vi "自动界面.vi"(8 "错误输入（无错误）":errorcluster, 10 "界面切换队列":refnum<queue>, 11 "VISA资源名称输入":refnum<visa-resource-name>) -> (0 "错误输出":errorcluster, 3 "VISA资源名称输出":refnum<visa-resource-name>)   [LabVIEW 2018]
panel:
  out "毫秒计时值":u32
  in  "枚举":T1(ring)
  in  "选项卡控件":enum32{"选项卡 1", "选项卡 2"}(tab)
  in  "报警显示":string
  out "写R2490":bool
  out "写R80":bool
  out "写R9+读R8":bool
  out "写R6+读R7":bool
  out "写R88+读R89":bool
  out "写R453":bool
  out "写R452":bool
  out "RF":bool
  out "DT1215":enum16{"关闭", "空", "烧录", "OK", "", "NG"}(ring)
  out "DT1211":enum16{"关闭", "空", "烧录", "OK", "", "NG"}(ring)
  out "DT1207":enum16{"关闭", "空", "烧录", "OK", "", "NG"}(ring)
  out "DT1203":enum16{"关闭", "空", "烧录", "OK", "", "NG"}(ring)
  out "DT1214":enum16{"关闭", "空", "烧录", "OK", "", "NG"}(ring)
  out "DT1210":enum16{"关闭", "空", "烧录", "OK", "", "NG"}(ring)
  out "DT1206":enum16{"关闭", "空", "烧录", "OK", "", "NG"}(ring)
  out "DT1202":enum16{"关闭", "空", "烧录", "OK", "", "NG"}(ring)
  out "DT1213":enum16{"关闭", "空", "烧录", "OK", "", "NG"}(ring)
  out "DT1209":enum16{"关闭", "空", "烧录", "OK", "", "NG"}(ring)
  out "DT1205":enum16{"关闭", "空", "烧录", "OK", "", "NG"}(ring)
  out "DT1201":enum16{"关闭", "空", "烧录", "OK", "", "NG"}(ring)
  out "DT1212":enum16{"关闭", "空", "烧录", "OK", "", "NG"}(ring)
  out "DT1208":enum16{"关闭", "空", "烧录", "OK", "", "NG"}(ring)
  out "DT1204":enum16{"关闭", "空", "烧录", "OK", "", "NG"}(ring)
  out "DT1200":enum16{"关闭", "空", "烧录", "OK", "", "NG"}(ring)
  out "R77":bool
  out "R76":bool
  out "R75":bool
  out "DT776":dbl
  out "DT770":dbl
  out "DT676":dbl
  out "DT670":dbl
  out "DT666":dbl
  out "DT660":dbl
  out "DDT594":dbl
  out "DDT604":dbl
  out "DDT600":dbl
  out "DDT590":dbl
  out "DDT32700":dbl
  out "DDT32750":dbl
  out "DDT32748":dbl
  out "DT1000+6位":string
  out "DT32622":dbl
  out "DDT90356":dbl
  out "DDT90348":dbl
  out "自动界面":bool
  out "手动界面":bool
  out "参数界面":bool
  out "IO界面":bool
  out "产品界面":bool
  out "字符串":string
  out "DDT90352":dbl
  out "DDT90360":dbl
  out "XC":bool
  out "写R454":bool
  out "写R2+读R3":bool
  out "写R87":bool
  out "通讯周期":dbl
  out "DT1184":T2(ring)
  # "X"
  # "Z1"
  # "Z2"
  # "Y"
  # "设定产量"
  # "当前产品"
  # "当前产量"
  # "NG产量"
  # "烧录座状态"
  # "修改"
  # "已取"
  # "行数"
  # "列数"
  # "已放"
  # "04"
  # "03"
  # "主料盘"
  # "02"
  # "01"
  # "08"
  # "07"
  # "05"
  # "06"
  # "备料盘"
  # "12"
  # "11"
  # "09"
  # "10"
  # "废料盘"
  # "14"
  # "15"
  # "13"
  # "14"
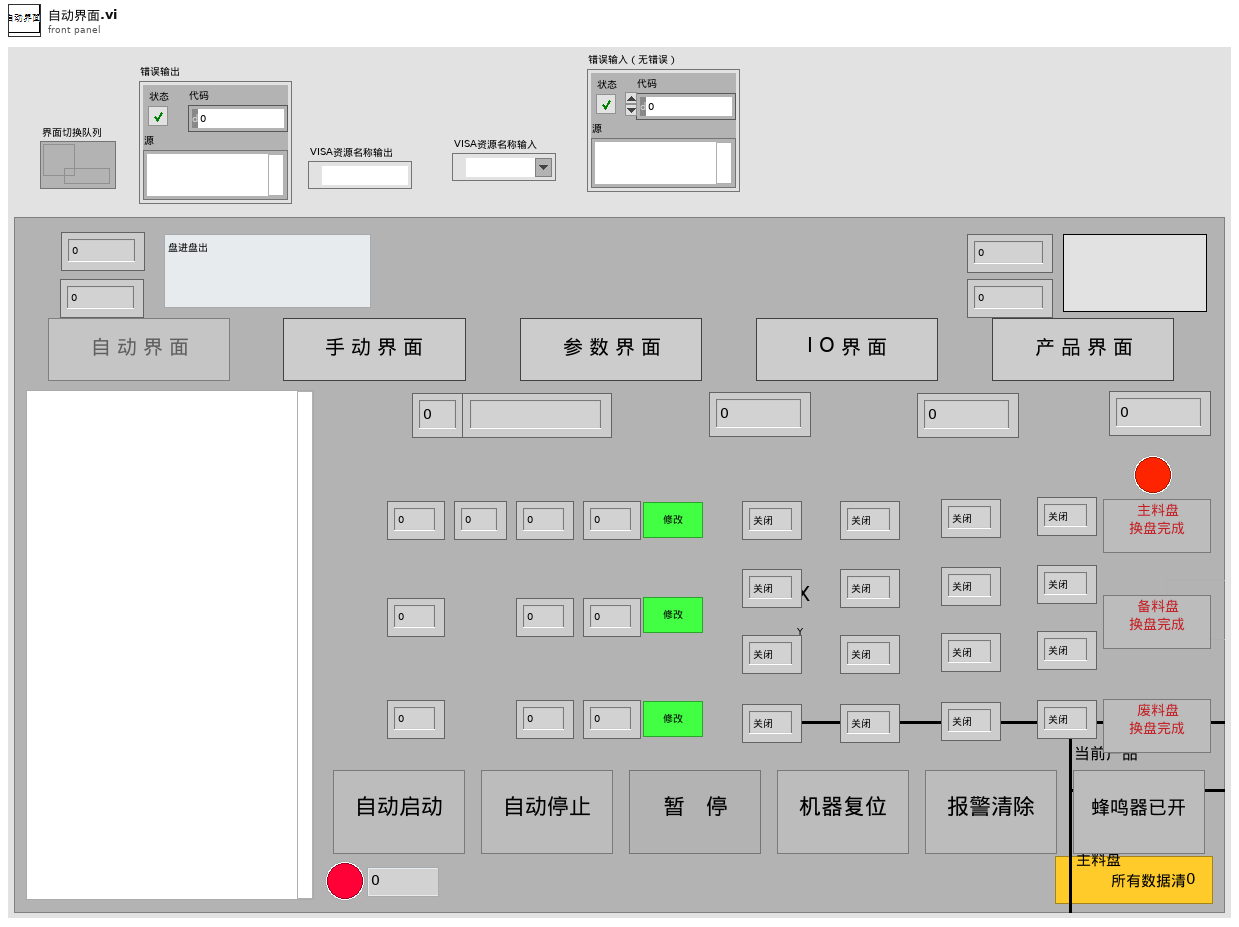
[diagram p1: front panel]
types:
  T1 = enum16{"读初始化", "读R598+8+报警", "读R590+8+报警", "读R588+8+报警", "读R580+8+报警", "读R405+8+报警", "读R410+8+报警", "读R221+8+报警", "读R449+8+报警", "读R450+8+报警", "读R441+8+报警", "读R89+8+报警", "读R72+8+报警", "读X1C+8+报警", "读R400+8+报警", "读T700+8+报警", "读X8+8+报警", "读R80+8", "读RF+8", "读XC+8", "读R2490+8", "读R452+8", "读R87+8", "读R75+8", "读R2+8", "读DDT90356", "读DT1184", "读DT1000+6", "读DT1210+10", "读DT1200+10", "读DT770", "读DT32622", "无", "读DDT32700", "读DDT32750+10", "读DT670+10", "读DT660+10", "读DDT600+10", "读DDT590+10", "读DDT90348", ""}
  T2 = enum16{"盘进盘出", "卷进卷出", "盘进卷出", "管进盘出", "管进卷出", "卷进盘出", ""}
  T3 = enum8{"Enabled", "Disabled", "Disabled and Grayed Out"}
  T4 = typedef "数据簇.ctl" = cluster{"字符串":string, "数值":i32, "布尔":bool}
  T5 = typedef "lveventtype.ctl" = enum32{"Null", "Timeout", "Annotation Menu Selection", "Annotation Menu Selection?", "App Instance Close", "App Instance Close?", "Autoscale Range Change", "Bookmark Info Change", "Cell Edit", "Cell Edit?", "Cursor Grab", "Cursor Grab?", "Cursor Menu Selection", "Cursor Menu Selection?", "Cursor Move", "Cursor Release", "Data Change", "Direction Change", "Display State Change", "Drag Ended", "Drag Enter", "Drag Leave", "Drag Over", "Drag Source Update", "Drag Starting", "Drag Starting?", "Drop", "Exec State Change", "Key Down", "Key Down?", "Key Repeat", "Key Repeat?", "Key Up", "Listbox Double Click", "Menu Activation?", "Menu Selection (App)", "Menu Selection? (App)", "Menu Selection (User)", "Mouse Down", "Mouse Down?", "Mouse Enter", "Mouse Leave", "Mouse Move", "Mouse Up", "Mouse Wheel", "NI Security User Change (App)", "Pane Size", "Panel Close", "Panel Close?", "Panel Resize", "Plot Attribute Change", "Scale Range Change", "Shortcut Menu Activation?", "Shortcut Menu Selection (App)", "Shortcut Menu Selection? (App)", "Shortcut Menu Selection (User)", "Tree Double Click", "Tree Drag", "Tree Drag?", "Tree Drop", "Tree Drop?", "Tree Item Close", "Tree Item Close?", "Tree Item Open", "Tree Item Open?", "User Event", "Value Change"}
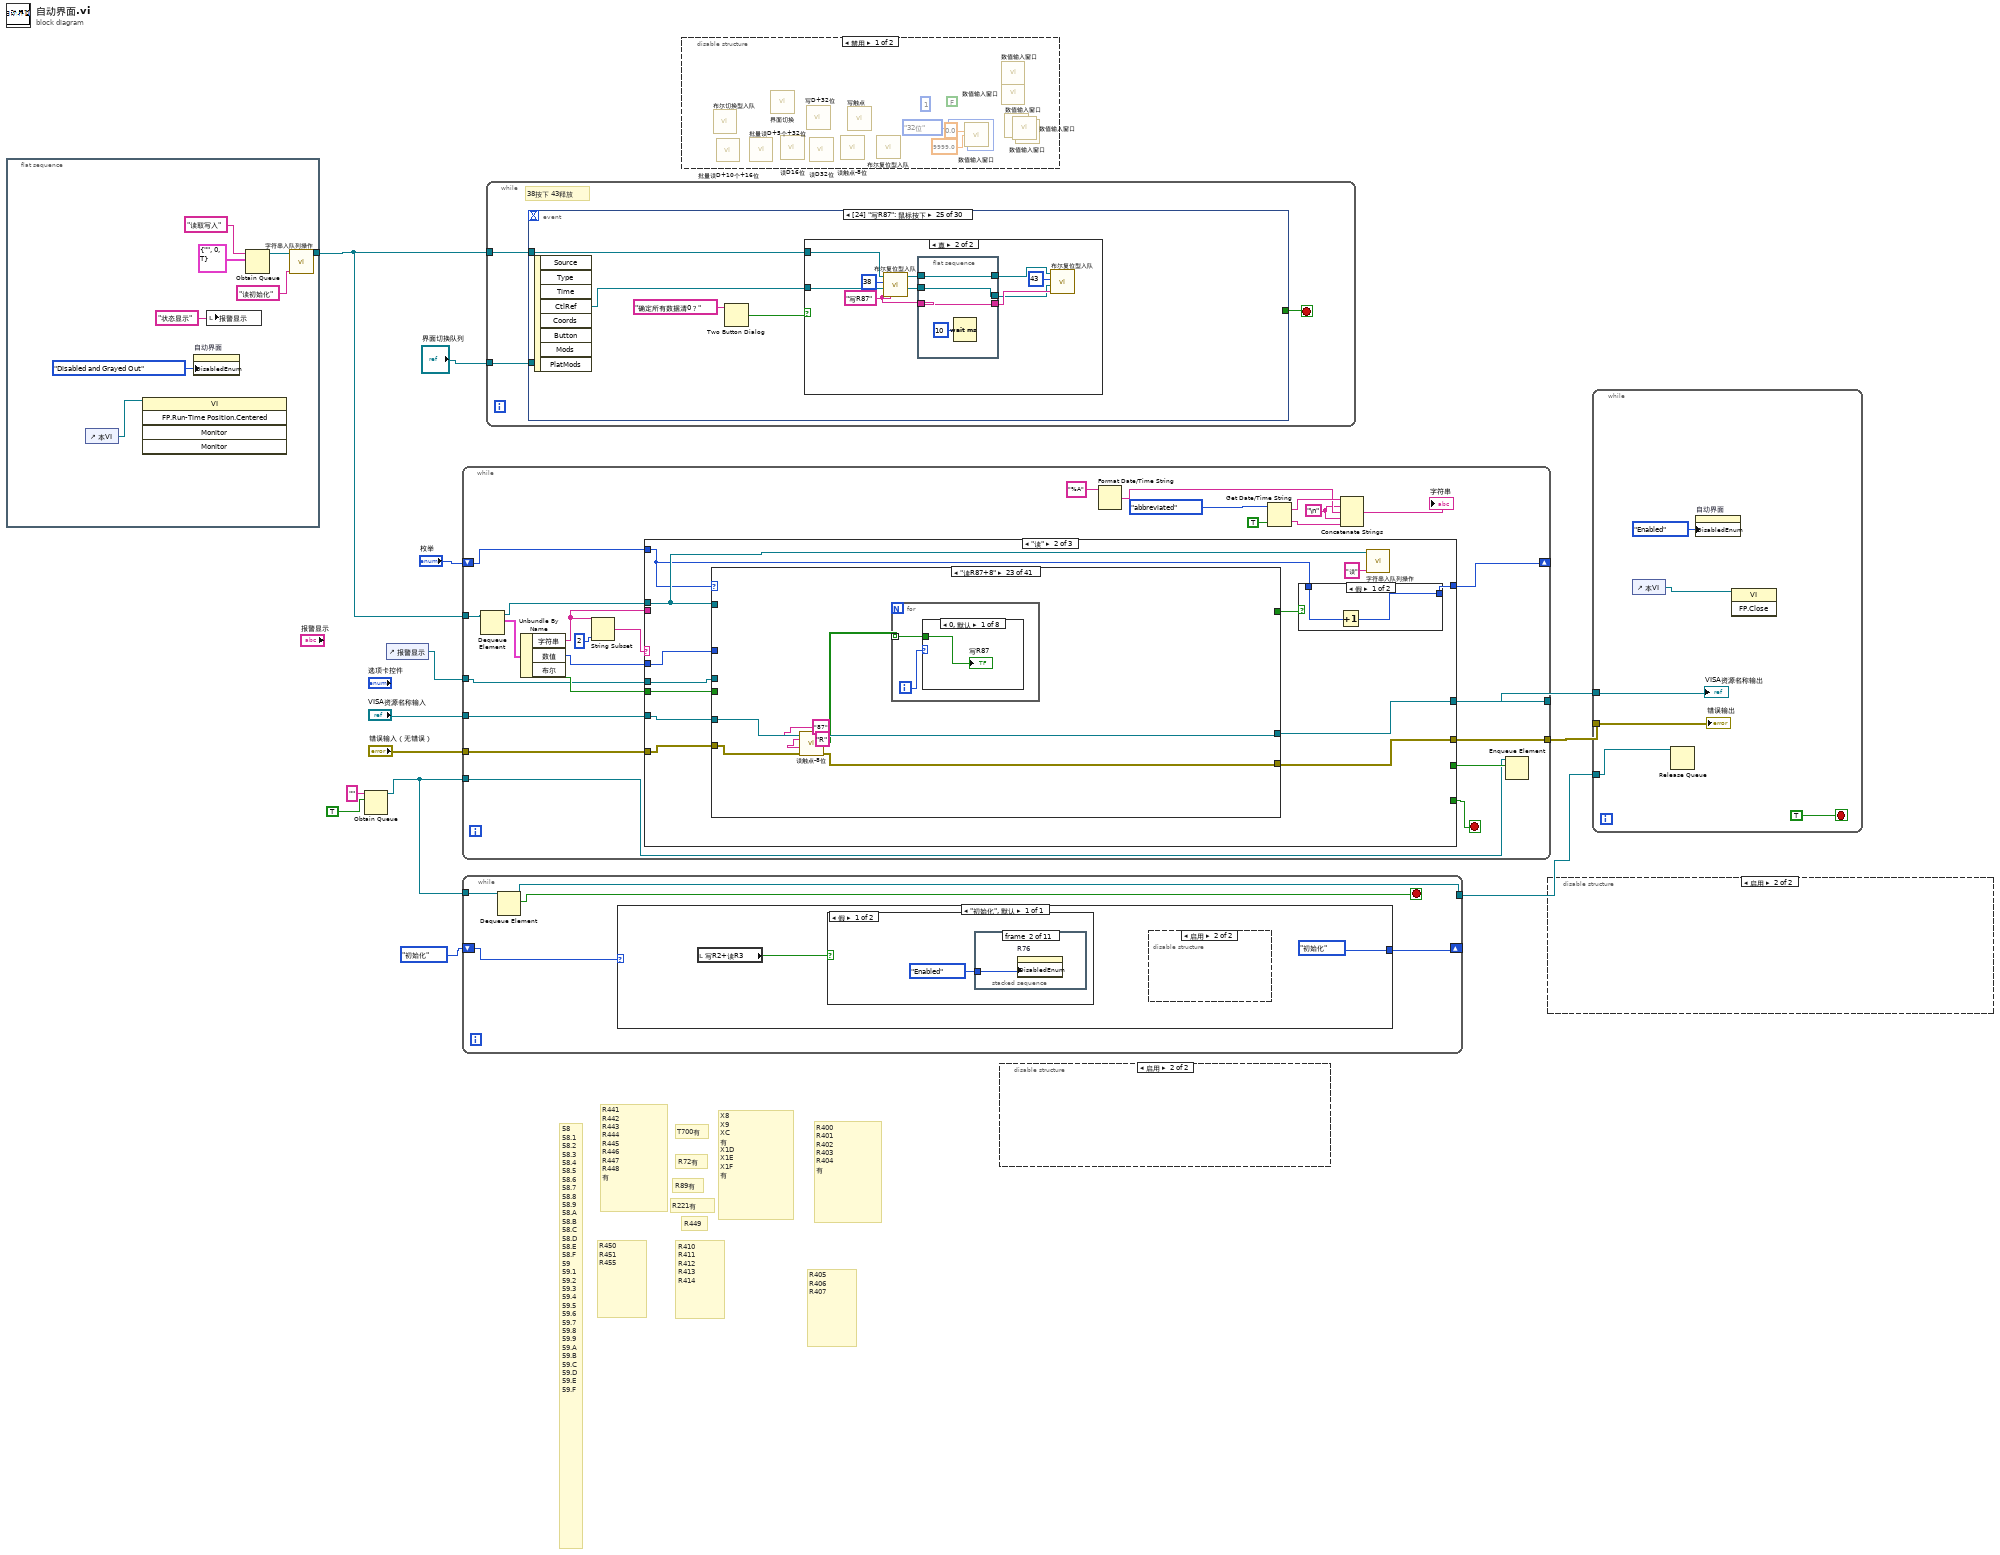
[diagram p0: block diagram]
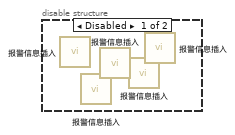
[diagram p2: hidden frame]
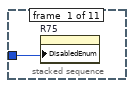
[diagram p3: hidden frame]
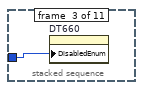
[diagram p4: hidden frame]
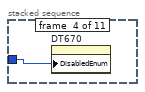
[diagram p5: hidden frame]
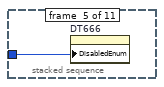
[diagram p6: hidden frame]
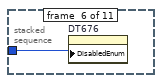
[diagram p7: hidden frame]
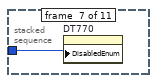
[diagram p8: hidden frame]
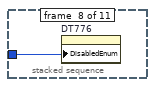
[diagram p9: hidden frame]
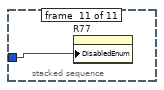
[diagram p12: hidden frame]
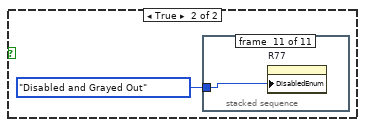
[diagram p13: hidden frame]
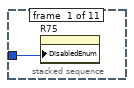
[diagram p14: hidden frame]
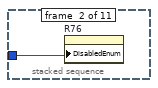
[diagram p15: hidden frame]
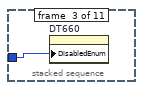
[diagram p16: hidden frame]
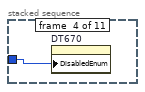
[diagram p17: hidden frame]
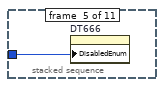
[diagram p18: hidden frame]
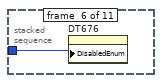
[diagram p19: hidden frame]
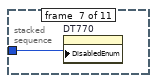
[diagram p20: hidden frame]
diagram:
  # "R449"
  # "R405\nR406\nR407"
  # "R410\nR411\nR412\nR413\nR414"
  # "R221有"
  # "R89有"
  # "R450\nR451\nR455"
  # "R72有"
  # "R441\nR442\nR443\nR444\nR445\nR446\nR447\nR448\n有"
  # "R400\nR401\nR402\nR403\nR404\n有"
  # "T700有"
  # "X8\nX9\nXC\n有\nX1D\nX1E\nX1F\n有"
  # "58\n58.1\n58.2\n58.3\n58.4\n58.5\n58.6\n58.7\n58.8\n58.9\n58.A\n58.B\n58.C\n58.D\n58.E\n58.F\n59\n59.1\n59.2\n59.3\n59.4\n59.5\n59.6\n59.7\n59.8\n59.9\n59.A\n59.B\n59.C\n59.D\n59.E\n59.F"
  n1 = flat-sequence {
    tunnel: [w21] -> w2
    frame #0 {
      n2 = control-ref of="本VI"() -> (w14:refnum<vi>)
      n3 = invoke class="VI" method="FP.Run-Time Position.Centered"(reference=w14) -> ()  [unwired: 4 in, 5 out]
      n4 = property on="自动界面" class="Bool"("DisabledEnum"=T3."Disabled and Grayed Out" ("禁用")) -> ()  [unwired: 2 in, 2 out]
      n5 = local write "报警显示"("状态显示") -> ()
      n6 = Obtain Queue(name (unnamed)="读取写入" ("名称（未命名）"), element data type=T4 {"字符串"="", "数值"=0, "布尔"=TRUE}) -> (queue out=w17:refnum<queue>)  [unwired: 3 in, 2 out]
      n7 = call "字符串入队列操作.vi"("字符消息入队列"="读初始化", "界面切换队列"=w17) -> ("队列输出"=w21:refnum<queue>)  [unwired: 9 in]
    }
  }
  n8 = Obtain Queue(name (unnamed)="" ("名称（未命名）"), element data type=TRUE) -> (queue out=w6:refnum<queue>)  [unwired: 3 in, 2 out]
  n9 = control-ref of="报警显示"() -> (w4:refnum<vi>)
  n10 = while {
    tunnel: w2 -> [w43]
    tunnel: "VISA资源名称输入" -> [w36]
    tunnel: "错误输入（无错误）" -> [w35]
    tunnel: [w34] -> w11
    tunnel: [w33] -> w10
    shift-right: [w30] -> _
    shift-left: "枚举" -> [w31]
    tunnel: w6 -> [w23]
    tunnel: w4 -> [w22]
    stop <- w25 stop-if-true
    w27 = "\n"
    n11 = Dequeue Element(queue=w43) -> (queue out=w40:refnum<queue>, element=w42:T4)  [unwired: 2 in, 2 out]
    n12 = Unbundle By Name(w42) -> ("字符串"=w37:string, "数值"=w39:i32, "布尔"=w38:bool)
    n13 = String Subset(string=w37, length (rest)=2 ("长度（剩余）")) -> (substring=w41:string)  [unwired: 1 in]
    n14 = case shown="\"读\"" w41 {
      selector: w41 -> [w50 _ _]
      tunnel: w40 -> [_ w59 w800]
      tunnel: w39 -> [_ w66 w799]
      tunnel: w38 -> [_ w65 w798]
      tunnel: w37 -> [_ _ w792]
      tunnel: w36 -> [w49 w64 w797]
      tunnel: w35 -> [w48 w63 w796]
      tunnel: [w49 w62 w794] -> w34
      tunnel: [w48 w61 w793] -> w33
      tunnel: [_ _ w795] -> w25
      tunnel: w31 -> [_ w57 _]
      tunnel: [_ w56 _] -> w30
      tunnel: [_ _ w790] -> w24
      tunnel: w22 -> [_ w55 _]
      frame "", Default {
        n15 = Concatenate Strings("无对应消息分支**" ("消息"), w50, "**" ("字符串"), "读写状态机" ("字符串")) -> (w52:string)
        n16 = One Button Dialog(message=w52) -> ()  [unwired: 1 in, 1 out]
      }
      frame "读" {
        n17 = case shown="\"读R87+8\"" w57 {
          tunnel: w59 -> [_ _ _ _ _ _ _ _ _ _ _ _ _ _ _ _ _ _ _ _ _ _ _ _ _ _ _ _ _ _ _ _ _ _ _ _ _ _ _ _ _]
          tunnel: w66 -> [_ _ _ _ _ _ _ _ _ _ _ _ _ _ _ _ _ _ _ _ _ _ _ _ _ _ _ _ _ _ _ _ _ _ _ _ _ _ _ _ _]
          tunnel: w64 -> [w71 w79 w117 w155 w193 w225 w236 w262 w284 w306 w330 w359 w381 w403 w431 w460 w491 w524 w534 w545 w556 w566 w578 w589 w601 w618 w627 w636 w665 w679 w697 w707 w709 w715 w721 w731 w741 w751 w761 w777 w789]
          tunnel: w63 -> [w70 w78 w116 w154 w192 w224 w235 w261 w283 w305 w329 w358 w380 w402 w430 w459 w490 w523 w533 w544 w555 w565 w577 w588 w600 w617 w626 w635 w664 w678 w696 w706 w708 w714 w720 w730 w740 w750 w760 w776 w788]
          tunnel: [w71 w75 w113 w151 w191 w225 w234 w260 w282 w304 w326 w355 w377 w399 w429 w456 w489 w520 w532 w541 w552 w562 w574 w585 w597 w616 w625 w629 w662 w676 w694 w704 w709 w712 w718 w728 w738 w749 w758 w775 w789] -> w62
          tunnel: [w70 w74 w112 w150 w190 w224 w233 w259 w281 w303 w325 w354 w376 w398 w428 w455 w488 w519 w531 w540 w551 w561 w573 w584 w596 w615 w624 w631 w661 w675 w693 w703 w708 w711 w717 w727 w737 w748 w757 w774 w788] -> w61
          tunnel: w65 -> [_ _ _ _ _ _ _ _ _ _ _ _ _ _ _ _ _ _ _ _ _ _ _ _ _ _ _ _ _ _ _ _ _ _ _ _ _ _ _ _ _]
          tunnel: [_ _ _ _ _ _ _ _ _ _ _ _ _ _ _ _ _ _ _ _ _ _ _ _ _ _ _ _ _ _ _ _ _ _ _ _ _ _ _ _ TRUE] -> w58
          tunnel: w55 -> [_ w72 w110 w148 w186 _ w229 w255 w277 w299 w323 w352 w374 w396 w424 w453 w484 _ _ w538 _ _ _ _ _ _ _ _ _ _ _ _ _ _ _ _ _ _ _ _ _]
          frame "读初始化" {
            n18 = Tick Count (ms)() -> (millisecond timer value=→"毫秒计时值":u32)
          }
          frame "读R598+8+报警" {
            n19 = call "读触点-8位.vi"("error out"=w78, "触点类型"="R", "读取起始地址"="598", "VISA resource name out"=w79) -> ("error IO"=w74:errorcluster, "读取布尔数组"=w73:bool[], "VISA resource name out 2"=w75:refnum<visa-resource-name>)  [unwired: 4 in, 1 out]
            n20 = for {
              tunnel: w73 -> [w84] mode=indexing
              tunnel: w72 -> [w83]
              i -> [w85]
              n21 = case shown="7" w85 {
                tunnel: w84 -> [w87 w90 w93 w96 w99 w102 w105 w108]
                tunnel: w83 -> [w88 w91 w94 w97 w100 w103 w106 w109]
                tunnel: [w88 w91 w94 w97 w100 w103 w106 w109] -> w82
                tunnel: [w87 w90 w93 w96 w99 w102 w105 w108] -> w81
                tunnel: ["9#烧录座连续NG超过设定的次数" "10#烧录座连续NG超过设定的次数" "11#烧录座连续NG超过设定的次数" "12#烧录座连续NG超过设定的次数" "13#烧录座连续NG超过设定的次数" "14#烧录座连续NG超过设定的次数" "15#烧录座连续NG超过设定的次数" "16#烧录座连续NG超过设定的次数"] -> w80
                frame 0, Default {
                }
                frame 1 {
                }
                frame 2 {
                }
                frame 3 {
                }
                frame 4 {
                }
                frame 5 {
                }
                frame 6 {
                }
                frame 7 {
                }
              }
              n22 = call "报警信息插入.vi"("输入字符串"=w80, "布尔"=w81, "Str引用句柄"=w82) -> ()  [unwired: 4 in, 1 out]
            }
          }
          frame "读R590+8+报警" {
            n23 = call "读触点-8位.vi"("error out"=w116, "触点类型"="R", "读取起始地址"="590", "VISA resource name out"=w117) -> ("error IO"=w112:errorcluster, "读取布尔数组"=w111:bool[], "VISA resource name out 2"=w113:refnum<visa-resource-name>)  [unwired: 4 in, 1 out]
            n24 = for {
              tunnel: w111 -> [w122] mode=indexing
              tunnel: w110 -> [w121]
              i -> [w123]
              n25 = case shown="7" w123 {
                tunnel: w122 -> [w125 w129 w131 w134 w137 w140 w143 w146]
                tunnel: w121 -> [w124 w128 w132 w135 w138 w141 w144 w147]
                tunnel: ["1#烧录座连续NG超过设定的次数" ("输入字符串") "2#烧录座连续NG超过设定的次数" ("输入字符串") "3#烧录座连续NG超过设定的次数" ("输入字符串") "4#烧录座连续NG超过设定的次数" ("输入字符串") "5#烧录座连续NG超过设定的次数" ("输入字符串") "6#烧录座连续NG超过设定的次数" ("输入字符串") "7#烧录座连续NG超过设定的次数" ("输入字符串") "8#烧录座连续NG超过设定的次数" ("输入字符串")] -> w120
                tunnel: [w125 w129 w131 w134 w137 w140 w143 w146] -> w119
                tunnel: [w124 w128 w132 w135 w138 w141 w144 w147] -> w118
                frame 0, Default {
                }
                frame 1 {
                }
                frame 2 {
                }
                frame 3 {
                }
                frame 4 {
                }
                frame 5 {
                }
                frame 6 {
                }
                frame 7 {
                }
              }
              n26 = call "报警信息插入.vi"("输入字符串"=w120, "布尔"=w119, "Str引用句柄"=w118) -> ()  [unwired: 4 in, 1 out]
            }
          }
          frame "读R588+8+报警" {
            n27 = call "读触点-8位.vi"("error out"=w154, "触点类型"="R", "读取起始地址"="588", "VISA resource name out"=w155) -> ("error IO"=w150:errorcluster, "读取布尔数组"=w149:bool[], "VISA resource name out 2"=w151:refnum<visa-resource-name>)  [unwired: 4 in, 1 out]
            n28 = for {
              tunnel: w149 -> [w160] mode=indexing
              tunnel: w148 -> [w159]
              i -> [w161]
              n29 = case shown="7" w161 {
                tunnel: w160 -> [w163 w166 w169 w172 w175 w178 w181 w184]
                tunnel: w159 -> [w164 w167 w170 w173 w176 w179 w182 w185]
                tunnel: [w164 w167 w170 w173 w176 w179 w182 w185] -> w158
                tunnel: [w163 w166 w169 w172 w175 w178 w181 w184] -> w157
                tunnel: ["9#烧录座到达设的的使用寿命" "10#烧录座到达设的的使用寿命" "11#烧录座到达设的的使用寿命" "12#烧录座到达设的的使用寿命" "13#烧录座到达设的的使用寿命" "14#烧录座到达设的的使用寿命" "15#烧录座到达设的的使用寿命" "16#烧录座到达设的的使用寿命"] -> w156
                frame 0, Default {
                }
                frame 1 {
                }
                frame 2 {
                }
                frame 3 {
                }
                frame 4 {
                }
                frame 5 {
                }
                frame 6 {
                }
                frame 7 {
                }
              }
              n30 = call "报警信息插入.vi"("输入字符串"=w156, "布尔"=w157, "Str引用句柄"=w158) -> ()  [unwired: 4 in, 1 out]
            }
          }
          frame "读R580+8+报警" {
            n31 = call "读触点-8位.vi"("error out"=w192, "触点类型"="R", "读取起始地址"="580", "VISA resource name out"=w193) -> ("error IO"=w190:errorcluster, "读取布尔数组"=w187:bool[], "VISA resource name out 2"=w191:refnum<visa-resource-name>)  [unwired: 4 in, 1 out]
            n32 = for {
              tunnel: w187 -> [w198] mode=indexing
              tunnel: w186 -> [w197]
              i -> [w199]
              n33 = case shown="7" w199 {
                tunnel: w198 -> [w201 w204 w207 w210 w213 w216 w219 w222]
                tunnel: w197 -> [w202 w205 w208 w211 w214 w217 w220 w223]
                tunnel: [w202 w205 w208 w211 w214 w217 w220 w223] -> w196
                tunnel: [w201 w204 w207 w210 w213 w216 w219 w222] -> w195
                tunnel: ["1#烧录座到达设的的使用寿命" "2#烧录座到达设的的使用寿命" "3#烧录座到达设的的使用寿命" "4#烧录座到达设的的使用寿命" "5#烧录座到达设的的使用寿命" "6#烧录座到达设的的使用寿命" "7#烧录座到达设的的使用寿命" "8#烧录座到达设的的使用寿命"] -> w194
                frame 0, Default {
                }
                frame 1 {
                }
                frame 2 {
                }
                frame 3 {
                }
                frame 4 {
                }
                frame 5 {
                }
                frame 6 {
                }
                frame 7 {
                }
              }
              n34 = call "报警信息插入.vi"("输入字符串"=w194, "布尔"=w195, "Str引用句柄"=w196) -> ()  [unwired: 4 in, 1 out]
            }
          }
          frame "读R405+8+报警" {
            n35 = disable-structure shown="禁用" {
              frame Disabled {
                (unwired) "R" ("触点类型")
                n36 = call "读触点-8位.vi"("读取起始地址"="405") -> ()  [unwired: 7 in, 4 out]
                n37 = for {
                  tunnel: _ -> [w227] mode=indexing
                  i -> [w228]
                  n38 = case shown="7" w228 {
                    tunnel: w227 -> [_ _ _ _ _ _ _ _]
                    frame 0, Default {
                    }
                    frame 1 {
                    }
                    frame 2 {
                    }
                    frame 3 {
                    }
                    frame 4 {
                    }
                    frame 5 {
                    }
                    frame 6 {
                    }
                    frame 7 {
                    }
                  }
                }
              }
              frame Enabled {
              }
            }
          }
          frame "读R410+8+报警" {
            n39 = call "读触点-8位.vi"("error out"=w235, "触点类型"="R", "读取起始地址"="410", "VISA resource name out"=w236) -> ("error IO"=w233:errorcluster, "读取布尔数组"=w230:bool[], "VISA resource name out 2"=w234:refnum<visa-resource-name>)  [unwired: 4 in, 1 out]
            n40 = for {
              tunnel: w230 -> [w240] mode=indexing
              tunnel: w229 -> [w239]
              i -> [w241]
              n41 = case shown="4" w241 {
                tunnel: w240 -> [w243 w245 w247 w249 w251 w252 w253 w254]
                tunnel: [w243 w245 w247 w249 w251 w252 w253 w254] -> w238
                tunnel: ["请给管道加料！" "X轴极限报警" "Y轴极限报警" "Z1轴极限报警" "Z2轴极限报警" _ _ _] -> w237
                frame 0, Default {
                }
                frame 1 {
                }
                frame 2 {
                }
                frame 3 {
                }
                frame 4 {
                }
                frame 5 {
                }
                frame 6 {
                }
                frame 7 {
                }
              }
              n42 = call "报警信息插入.vi"("输入字符串"=w237, "布尔"=w238, "Str引用句柄"=w239) -> ()  [unwired: 4 in, 1 out]
            }
          }
          frame "读R221+8+报警" {
            n43 = call "读触点-8位.vi"("error out"=w261, "触点类型"="R", "读取起始地址"="221", "VISA resource name out"=w262) -> ("error IO"=w259:errorcluster, "读取布尔数组"=w256:bool[], "VISA resource name out 2"=w260:refnum<visa-resource-name>)  [unwired: 4 in, 1 out]
            n44 = for {
              tunnel: w256 -> [w266] mode=indexing
              tunnel: w255 -> [w265]
              i -> [w267]
              n45 = case shown="0, 默认" w267 {
                tunnel: w266 -> [w269 w270 w271 w272 w273 w274 w275 w276]
                tunnel: [w269 w270 w271 w272 w273 w274 w275 w276] -> w264
                tunnel: ["正在待机！" _ _ _ _ _ _ _] -> w263
                frame 0, Default {
                }
                frame 1 {
                }
                frame 2 {
                }
                frame 3 {
                }
                frame 4 {
                }
                frame 5 {
                }
                frame 6 {
                }
                frame 7 {
                }
              }
              n46 = call "报警信息插入.vi"("输入字符串"=w263, "布尔"=w264, "Str引用句柄"=w265) -> ()  [unwired: 4 in, 1 out]
            }
          }
          frame "读R449+8+报警" {
            n47 = call "读触点-8位.vi"("error out"=w283, "触点类型"="R", "读取起始地址"="449", "VISA resource name out"=w284) -> ("error IO"=w281:errorcluster, "读取布尔数组"=w278:bool[], "VISA resource name out 2"=w282:refnum<visa-resource-name>)  [unwired: 4 in, 1 out]
            n48 = for {
              tunnel: w278 -> [w288] mode=indexing
              tunnel: w277 -> [w287]
              i -> [w289]
              n49 = case shown="0, 默认" w289 {
                tunnel: w288 -> [w291 w292 w293 w294 w295 w296 w297 w298]
                tunnel: [w291 w292 w293 w294 w295 w296 w297 w298] -> w286
                tunnel: ["没有收到卷带收料完成信号！R449" _ _ _ _ _ _ _] -> w285
                frame 0, Default {
                }
                frame 1 {
                }
                frame 2 {
                }
                frame 3 {
                }
                frame 4 {
                }
                frame 5 {
                }
                frame 6 {
                }
                frame 7 {
                }
              }
              n50 = call "报警信息插入.vi"("输入字符串"=w285, "布尔"=w286, "Str引用句柄"=w287) -> ()  [unwired: 4 in, 1 out]
            }
          }
          frame "读R450+8+报警" {
            n51 = call "读触点-8位.vi"("error out"=w305, "触点类型"="R", "读取起始地址"="450", "VISA resource name out"=w306) -> ("error IO"=w303:errorcluster, "读取布尔数组"=w300:bool[], "VISA resource name out 2"=w304:refnum<visa-resource-name>)  [unwired: 4 in, 1 out]
            n52 = for {
              tunnel: w300 -> [w310] mode=indexing
              tunnel: w299 -> [w309]
              i -> [w311]
              n53 = case shown="7" w311 {
                tunnel: w310 -> [w313 w315 w316 w317 w318 w320 w321 w322]
                tunnel: [w313 w315 w316 w317 w318 w320 w321 w322] -> w308
                tunnel: ["已完成设定的编带数量，要再次启动，请先将已完成数量清零！" "备料盘已取完，请更换备料盘，然后点击备料盘更换完成！" _ _ _ "NG数量到达提示数量，请注意！" _ _] -> w307
                frame 0, Default {
                }
                frame 1 {
                }
                frame 2 {
                }
                frame 3 {
                }
                frame 4 {
                }
                frame 5 {
                }
                frame 6 {
                }
                frame 7 {
                }
              }
              n54 = call "报警信息插入.vi"("输入字符串"=w307, "布尔"=w308, "Str引用句柄"=w309) -> ()  [unwired: 4 in, 1 out]
            }
          }
          frame "读R441+8+报警" {
            n55 = call "读触点-8位.vi"("error out"=w329, "触点类型"="R", "读取起始地址"="441", "VISA resource name out"=w330) -> ("error IO"=w325:errorcluster, "读取布尔数组"=w324:bool[], "VISA resource name out 2"=w326:refnum<visa-resource-name>)  [unwired: 4 in, 1 out]
            n56 = for {
              tunnel: w324 -> [w334] mode=indexing
              tunnel: w323 -> [w333]
              i -> [w335]
              n57 = case shown="1" w335 {
                tunnel: w334 -> [w337 w339 w341 w343 w345 w347 w349 w351]
                tunnel: [w337 w339 w341 w343 w345 w347 w349 w351] -> w332
                tunnel: ["生产模式时没收到自动换盘完成信号，不能启动！" "正在等待换盘完成！" "主料盘数量不能为0，请修改参数！" "备料盘数量不能为0，请修改参数！" "废料盘数量不能为0，请修改参数！" "废料盘已放满，请更换废料盘，然后点击废料盘更换完成！" "正在等待换盘！" "没有收到卷带收料完成信号！R448"] -> w331
                frame 0, Default {
                }
                frame 1 {
                }
                frame 2 {
                }
                frame 3 {
                }
                frame 4 {
                }
                frame 5 {
                }
                frame 6 {
                }
                frame 7 {
                }
              }
              n58 = call "报警信息插入.vi"("输入字符串"=w331, "布尔"=w332, "Str引用句柄"=w333) -> ()  [unwired: 4 in, 1 out]
            }
          }
          frame "读R89+8+报警" {
            n59 = call "读触点-8位.vi"("error out"=w358, "触点类型"="R", "读取起始地址"="89", "VISA resource name out"=w359) -> ("error IO"=w354:errorcluster, "读取布尔数组"=w353:bool[], "VISA resource name out 2"=w355:refnum<visa-resource-name>)  [unwired: 4 in, 1 out]
            n60 = for {
              tunnel: w353 -> [w363] mode=indexing
              tunnel: w352 -> [w362]
              i -> [w364]
              n61 = case shown="0, 默认" w364 {
                tunnel: w363 -> [w366 w367 w368 w369 w370 w371 w372 w373]
                tunnel: [w366 w367 w368 w369 w370 w371 w372 w373] -> w361
                tunnel: ["正在准备停机！" _ _ _ _ _ _ _] -> w360
                frame 0, Default {
                }
                frame 1 {
                }
                frame 2 {
                }
                frame 3 {
                }
                frame 4 {
                }
                frame 5 {
                }
                frame 6 {
                }
                frame 7 {
                }
              }
              n62 = call "报警信息插入.vi"("输入字符串"=w360, "布尔"=w361, "Str引用句柄"=w362) -> ()  [unwired: 4 in, 1 out]
            }
          }
          frame "读R72+8+报警" {
            n63 = call "读触点-8位.vi"("error out"=w380, "触点类型"="R", "读取起始地址"="72", "VISA resource name out"=w381) -> ("error IO"=w376:errorcluster, "读取布尔数组"=w375:bool[], "VISA resource name out 2"=w377:refnum<visa-resource-name>)  [unwired: 4 in, 1 out]
            n64 = for {
              tunnel: w375 -> [w385] mode=indexing
              tunnel: w374 -> [w384]
              i -> [w386]
              n65 = case shown="0, 默认" w386 {
                tunnel: w385 -> [w388 w389 w390 w391 w392 w393 w394 w395]
                tunnel: [w388 w389 w390 w391 w392 w393 w394 w395] -> w383
                tunnel: ["请先复位，然后再启动！" _ _ _ _ _ _ _] -> w382
                frame 0, Default {
                }
                frame 1 {
                }
                frame 2 {
                }
                frame 3 {
                }
                frame 4 {
                }
                frame 5 {
                }
                frame 6 {
                }
                frame 7 {
                }
              }
              n66 = call "报警信息插入.vi"("输入字符串"=w382, "布尔"=w383, "Str引用句柄"=w384) -> ()  [unwired: 4 in, 1 out]
            }
          }
          frame "读X1C+8+报警" {
            n67 = call "读触点-8位.vi"("error out"=w402, "触点类型"="X", "读取起始地址"="1C", "VISA resource name out"=w403) -> ("error IO"=w398:errorcluster, "读取布尔数组"=w397:bool[], "VISA resource name out 2"=w399:refnum<visa-resource-name>)  [unwired: 4 in, 1 out]
            n68 = for {
              tunnel: w397 -> [w407] mode=indexing
              tunnel: w396 -> [w406]
              i -> [w408]
              n69 = case shown="3" w408 {
                tunnel: w407 -> [w410 w412 w415 w418 w420 w421 w422 w423]
                tunnel: [w410 w411 w414 w417 w420 w421 w422 w423] -> w405
                tunnel: ["X轴报警中！" "Y轴报警中！" "Z1轴报警中！" "Z2轴报警中！" _ _ _ _] -> w404
                frame 0, Default {
                }
                frame 1 {
                  n70 = Not(x=w412) -> (.not. x?=w411:bool)
                }
                frame 2 {
                  n71 = Not(x=w415) -> (.not. x?=w414:bool)
                }
                frame 3 {
                  n72 = Not(x=w418) -> (.not. x?=w417:bool)
                }
                frame 4 {
                }
                frame 5 {
                }
                frame 6 {
                }
                frame 7 {
                }
              }
              n73 = call "报警信息插入.vi"("输入字符串"=w404, "布尔"=w405, "Str引用句柄"=w406) -> ()  [unwired: 4 in, 1 out]
            }
          }
          frame "读R400+8+报警" {
            n74 = call "读触点-8位.vi"("error out"=w430, "触点类型"="R", "读取起始地址"="400", "VISA resource name out"=w431) -> ("error IO"=w428:errorcluster, "读取布尔数组"=w425:bool[], "VISA resource name out 2"=w429:refnum<visa-resource-name>)  [unwired: 4 in, 1 out]
            n75 = for {
              tunnel: w425 -> [w435] mode=indexing
              tunnel: w424 -> [w434]
              i -> [w436]
              n76 = case shown="7" w436 {
                tunnel: w435 -> [w438 w440 w442 w444 w446 w448 w450 w452]
                tunnel: [w438 w440 w442 w444 w446 w448 w450 w452] -> w433
                tunnel: ["1号吸嘴信号异常！" "2号吸嘴信号异常！" "Z1轴原点异常！" "Z2轴原点异常！" "Z1轴吸料失败！" "Z2轴吸料失败！" "1#吸嘴掉料报警中！" "2#吸嘴掉料报警中！"] -> w432
                frame 0, Default {
                }
                frame 1 {
                }
                frame 2 {
                }
                frame 3 {
                }
                frame 4 {
                }
                frame 5 {
                }
                frame 6 {
                }
                frame 7 {
                }
              }
              n77 = call "报警信息插入.vi"("输入字符串"=w432, "布尔"=w433, "Str引用句柄"=w434) -> ()  [unwired: 4 in, 1 out]
            }
          }
          frame "读T700+8+报警" {
            n78 = call "读触点-8位.vi"("error out"=w459, "触点类型"="T", "读取起始地址"="700", "VISA resource name out"=w460) -> ("error IO"=w455:errorcluster, "读取布尔数组"=w454:bool[], "VISA resource name out 2"=w456:refnum<visa-resource-name>)  [unwired: 4 in, 1 out]
            n79 = for {
              tunnel: w454 -> [w465] mode=indexing
              tunnel: w453 -> [w464]
              i -> [w466]
              n80 = case shown="1" w466 {
                tunnel: w465 -> [w468 w470 w472 w474 w476 w478 w480 w482]
                tunnel: [w469 w471 w473 w475 w477 w479 w481 w483] -> w463
                tunnel: w464 -> [w469 w471 w473 w475 w477 w479 w481 w483]
                tunnel: [w468 w470 w472 w474 w476 w478 w480 w482] -> w462
                tunnel: ["自动换盘超时！" _ _ _ _ _ _ _] -> w461
                frame 0, Default {
                }
                frame 1 {
                }
                frame 2 {
                }
                frame 3 {
                }
                frame 4 {
                }
                frame 5 {
                }
                frame 6 {
                }
                frame 7 {
                }
              }
              n81 = call "报警信息插入.vi"("输入字符串"=w461, "布尔"=w462, "Str引用句柄"=w463) -> ()  [unwired: 4 in, 1 out]
            }
          }
          frame "读X8+8+报警" {
            n82 = call "读触点-8位.vi"("error out"=w490, "触点类型"="X", "读取起始地址"="8", "VISA resource name out"=w491) -> ("error IO"=w488:errorcluster, "读取布尔数组"=w485:bool[], "VISA resource name out 2"=w489:refnum<visa-resource-name>)  [unwired: 4 in, 1 out]
            n83 = for {
              tunnel: w485 -> [w496] mode=indexing
              tunnel: w484 -> [w495]
              i -> [w497]
              n84 = case shown="0, 默认" w497 {
                tunnel: w496 -> [w499 w503 w506 w508 w510 w512 w514 w516]
                tunnel: [w501 w505 w507 w509 w511 w513 w515 w517] -> w494
                tunnel: w495 -> [w501 w505 w507 w509 w511 w513 w515 w517]
                tunnel: [w498 w502 w506 w508 w510 w512 w514 w516] -> w493
                tunnel: ["安全门打开中！" "急停中！" _ _ _ _ _ _] -> w492
                frame 0, Default {
                  n85 = Not(x=w499) -> (.not. x?=w498:bool)
                }
                frame 1 {
                  n86 = Not(x=w503) -> (.not. x?=w502:bool)
                }
                frame 2 {
                }
                frame 3 {
                }
                frame 4 {
                }
                frame 5 {
                }
                frame 6 {
                }
                frame 7 {
                }
              }
              n87 = call "报警信息插入.vi"("输入字符串"=w492, "布尔"=w493, "Str引用句柄"=w494) -> ()  [unwired: 4 in, 1 out]
            }
          }
          frame "读R80+8" {
            n88 = call "读触点-8位.vi"("error out"=w523, "触点类型"="R", "读取起始地址"="80", "VISA resource name out"=w524) -> ("error IO"=w519:errorcluster, "读取布尔数组"=w518:bool[], "VISA resource name out 2"=w520:refnum<visa-resource-name>)  [unwired: 4 in, 1 out]
            n89 = for {
              tunnel: w518 -> [w525] mode=indexing
              i -> [w526]
              n90 = case shown="0, 默认" w526 {
                tunnel: w525 -> [w527 _ _ _ _ _ _ _]
                frame 0, Default {
                  "写R80" <- w527
                }
                frame 1 {
                }
                frame 2 {
                }
                frame 3 {
                }
                frame 4 {
                }
                frame 5 {
                }
                frame 6 {
                }
                frame 7 {
                }
              }
            }
          }
          frame "读RF+8" {
            n91 = call "读触点-8位.vi"("error out"=w533, "触点类型"="R", "读取起始地址"="F", "VISA resource name out"=w534) -> ("error IO"=w531:errorcluster, "读取布尔数组"=w528:bool[], "VISA resource name out 2"=w532:refnum<visa-resource-name>)  [unwired: 4 in, 1 out]
            n92 = for {
              tunnel: w528 -> [w535] mode=indexing
              i -> [w536]
              n93 = case shown="0, 默认" w536 {
                tunnel: w535 -> [w537 _ _ _ _ _ _ _]
                frame 0, Default {
                  "RF" <- w537
                }
                frame 1 {
                }
                frame 2 {
                }
                frame 3 {
                }
                frame 4 {
                }
                frame 5 {
                }
                frame 6 {
                }
                frame 7 {
                }
              }
            }
          }
          frame "读XC+8" {
            n94 = call "读触点-8位.vi"("error out"=w544, "触点类型"="X", "读取起始地址"="1C", "VISA resource name out"=w545) -> ("error IO"=w540:errorcluster, "读取布尔数组"=w539:bool[], "VISA resource name out 2"=w541:refnum<visa-resource-name>)  [unwired: 4 in, 1 out]
            n95 = for {
              tunnel: w539 -> [w547] mode=indexing
              tunnel: w538 -> [w546]
              i -> [w548]
              n96 = case shown="1" w548 {
                tunnel: w547 -> [w549 _ _ _ _ _ _ _]
                tunnel: w546 -> [_ _ _ _ _ _ _ _]
                frame 0, Default {
                  "XC" <- w549
                }
                frame 1 {
                }
                frame 2 {
                }
                frame 3 {
                }
                frame 4 {
                }
                frame 5 {
                }
                frame 6 {
                }
                frame 7 {
                }
              }
            }
          }
          frame "读R2490+8" {
            n97 = call "读触点-8位.vi"("error out"=w555, "触点类型"="R", "读取起始地址"="2490", "VISA resource name out"=w556) -> ("error IO"=w551:errorcluster, "读取布尔数组"=w550:bool[], "VISA resource name out 2"=w552:refnum<visa-resource-name>)  [unwired: 4 in, 1 out]
            n98 = for {
              tunnel: w550 -> [w557] mode=indexing
              i -> [w558]
              n99 = case shown="0, 默认" w558 {
                tunnel: w557 -> [w559 _ _ _ _ _ _ _]
                frame 0, Default {
                  "写R2490" <- w559
                }
                frame 1 {
                }
                frame 2 {
                }
                frame 3 {
                }
                frame 4 {
                }
                frame 5 {
                }
                frame 6 {
                }
                frame 7 {
                }
              }
            }
          }
          frame "读R452+8" {
            n100 = call "读触点-8位.vi"("error out"=w565, "触点类型"="R", "读取起始地址"="452", "VISA resource name out"=w566) -> ("error IO"=w561:errorcluster, "读取布尔数组"=w560:bool[], "VISA resource name out 2"=w562:refnum<visa-resource-name>)  [unwired: 4 in, 1 out]
            n101 = for {
              tunnel: w560 -> [w567] mode=indexing
              i -> [w568]
              n102 = case shown="2" w568 {
                tunnel: w567 -> [w569 w570 w571 _ _ _ _ _]
                frame 0, Default {
                  "写R452" <- w569
                }
                frame 1 {
                  "写R453" <- w570
                }
                frame 2 {
                  "写R454" <- w571
                }
                frame 3 {
                }
                frame 4 {
                }
                frame 5 {
                }
                frame 6 {
                }
                frame 7 {
                }
              }
            }
          }
          frame "读R87+8" {
            n103 = call "读触点-8位.vi"("error out"=w577, "触点类型"="R", "读取起始地址"="87", "VISA resource name out"=w578) -> ("error IO"=w573:errorcluster, "读取布尔数组"=w572:bool[], "VISA resource name out 2"=w574:refnum<visa-resource-name>)  [unwired: 4 in, 1 out]
            n104 = for {
              tunnel: w572 -> [w579] mode=indexing
              i -> [w580]
              n105 = case shown="0, 默认" w580 {
                tunnel: w579 -> [w581 _ w582 _ _ _ _ _]
                frame 0, Default {
                  "写R87" <- w581
                }
                frame 1 {
                }
                frame 2 {
                  "写R88+读R89" <- w582
                }
                frame 3 {
                }
                frame 4 {
                }
                frame 5 {
                }
                frame 6 {
                }
                frame 7 {
                }
              }
            }
          }
          frame "读R75+8" {
            n106 = call "读触点-8位.vi"("error out"=w588, "触点类型"="R", "读取起始地址"="75", "VISA resource name out"=w589) -> ("error IO"=w584:errorcluster, "读取布尔数组"=w583:bool[], "VISA resource name out 2"=w585:refnum<visa-resource-name>)  [unwired: 4 in, 1 out]
            n107 = for {
              tunnel: w583 -> [w590] mode=indexing
              i -> [w591]
              n108 = case shown="2" w591 {
                tunnel: w590 -> [w592 w593 w594 _ _ _ _ _]
                frame 0, Default {
                  "R75" <- w592
                }
                frame 1 {
                  "R76" <- w593
                }
                frame 2 {
                  "R77" <- w594
                }
                frame 3 {
                }
                frame 4 {
                }
                frame 5 {
                }
                frame 6 {
                }
                frame 7 {
                }
              }
            }
          }
          frame "读R2+8" {
            n109 = call "读触点-8位.vi"("error out"=w600, "触点类型"="R", "读取起始地址"="2", "VISA resource name out"=w601) -> ("error IO"=w596:errorcluster, "读取布尔数组"=w595:bool[], "VISA resource name out 2"=w597:refnum<visa-resource-name>)  [unwired: 4 in, 1 out]
            n110 = for {
              tunnel: w595 -> [w602] mode=indexing
              i -> [w603]
              n111 = case shown="6" w603 {
                tunnel: w602 -> [_ w604 _ _ _ w605 w606 _]
                frame 0, Default {
                }
                frame 1 {
                  "写R2+读R3" <- w604
                }
                frame 2 {
                }
                frame 3 {
                }
                frame 4 {
                }
                frame 5 {
                  "写R6+读R7" <- w605
                }
                frame 6 {
                  "写R9+读R8" <- w606
                }
                frame 7 {
                }
              }
            }
          }
          frame "读DDT90356" {
            n112 = call "批量读D+5个+32位.vi"("error out"=w617, "读取D地址"=90356, "VISA resource name out"=w618) -> ("error IO"=w615:errorcluster, "数组"=w621:i32[], "VISA resource name out 2"=w616:refnum<visa-resource-name>)  [unwired: 5 in, 1 out]
            n113 = Index Array(array=w621, index #1=0 ("索引"), index #2=2 ("索引")) -> (element #1=w614:i32, element #2=w613:i32)
            n114 = To Double Precision Float(number=w614) -> (double precision float=w612:dbl)
            n115 = To Double Precision Float(number=w613) -> (double precision float=w609:dbl)
            n116 = Divide(x=w612, y=100.0) -> (x/y=→"DDT90356":dbl)
            n117 = Divide(x=w609, y=100.0) -> (x/y=→"DDT90360":dbl)
          }
          frame "读DT1184" {
            n118 = call "读D16位.vi"("error out"=w626, "读取D地址"=1184, "VISA resource name out"=w627) -> ("error IO"=w624:errorcluster, "数值"=→"DT1184":u32, "VISA resource name out 2"=w625:refnum<visa-resource-name>)  [unwired: 5 in, 1 out]
          }
          frame "读DT1000+6" {
            n119 = call "批量读D+10个+16位.vi"("error out"=w635, "读取D地址"=1000, "VISA resource name out"=w636) -> ("error IO"=w632:errorcluster, "读取缓冲区"=w633:string, "VISA resource name out 2"=w630:refnum<visa-resource-name>)  [unwired: 5 in, 1 out]
            n120 = case shown="无错误" w632 {
              selector: w632 -> [w638 w659]
              tunnel: w633 -> [w646 _]
              tunnel: [w638 w659] -> w631
              tunnel: [w637 w658] -> w629
              tunnel: w630 -> [w637 w658]
              frame No Error {
                n121 = String Subset(string=w646, offset (0)=6 ("偏移量(0)"), length (rest)=24 ("长度（剩余）")) -> (substring=w640:string)
                n122 = String Length(string=w640) -> (length=w645:i32)
                n123 = Divide(x=w645, y=2) -> (x/y=w643:dbl)
                n124 = for {
                  N: w643 -> [_]
                  shift-right: [w649] -> w639
                  shift-left: "" -> [w651]
                  tunnel: w640 -> [w657]
                  shift-right: [w653] -> _
                  shift-left: 0 -> [w652]
                  n125 = String Subset(string=w657, offset (0)=w652, length (rest)=2 ("长度（剩余）")) -> (substring=w656:string)
                  n126 = call "ascii转文本.vi"("输入"=w656) -> ("输出"=w650:string)  [unwired: 9 in, 1 out]
                  n127 = Concatenate Strings(w651, w650) -> (w649:string)
                  n128 = Add(x=w652, y=2) -> (x+y=w653:i32)
                }
                "DT1000+6位" <- w639
              }
              frame Error {
              }
            }
          }
          frame "读DT1210+10" {
            n129 = call "批量读D+10个+16位.vi"("error out"=w664, "读取D地址"=1210, "VISA resource name out"=w665) -> ("error IO"=w661:errorcluster, "数组"=w660:i32[], "VISA resource name out 2"=w662:refnum<visa-resource-name>)  [unwired: 5 in, 1 out]
            n130 = for {
              tunnel: w660 -> [w667] mode=indexing
              i -> [w666]
              n131 = case shown="4" w666 {
                tunnel: w667 -> [w668 w669 w670 w671 w672 w673 _ _ _ _]
                frame 0, Default {
                  "DT1210" <- w668
                }
                frame 1 {
                  "DT1211" <- w669
                }
                frame 2 {
                  "DT1212" <- w670
                }
                frame 3 {
                  "DT1213" <- w671
                }
                frame 4 {
                  "DT1214" <- w672
                }
                frame 5 {
                  "DT1215" <- w673
                }
                frame 6 {
                }
                frame 7 {
                }
                frame 8 {
                }
                frame 9 {
                }
              }
            }
          }
          frame "读DT1200+10" {
            n132 = call "批量读D+10个+16位.vi"("error out"=w678, "读取D地址"=1200, "VISA resource name out"=w679) -> ("error IO"=w675:errorcluster, "数组"=w674:i32[], "VISA resource name out 2"=w676:refnum<visa-resource-name>)  [unwired: 5 in, 1 out]
            n133 = for {
              tunnel: w674 -> [w681] mode=indexing
              i -> [w680]
              n134 = case shown="0, 默认" w680 {
                tunnel: w681 -> [w682 w683 w684 w685 w686 w687 w688 w689 w690 w691]
                frame 0, Default {
                  "DT1200" <- w682
                }
                frame 1 {
                  "DT1201" <- w683
                }
                frame 2 {
                  "DT1202" <- w684
                }
                frame 3 {
                  "DT1203" <- w685
                }
                frame 4 {
                  "DT1204" <- w686
                }
                frame 5 {
                  "DT1205" <- w687
                }
                frame 6 {
                  "DT1206" <- w688
                }
                frame 7 {
                  "DT1207" <- w689
                }
                frame 8 {
                  "DT1208" <- w690
                }
                frame 9 {
                  "DT1209" <- w691
                }
              }
            }
          }
          frame "读DT770" {
            n135 = call "批量读D+10个+16位.vi"("error out"=w696, "读取D地址"=770, "VISA resource name out"=w697) -> ("error IO"=w693:errorcluster, "数组"=w692:i32[], "VISA resource name out 2"=w694:refnum<visa-resource-name>)  [unwired: 5 in, 1 out]
            n136 = for {
              tunnel: w692 -> [w698] mode=indexing
              i -> [w699]
              n137 = case shown="5" w699 {
                tunnel: w698 -> [w700 _ _ _ _ _ w701 _ _ _]
                frame 0, Default {
                  "DT770" <- w700
                }
                frame 1 {
                }
                frame 2 {
                }
                frame 3 {
                }
                frame 4 {
                }
                frame 5 {
                }
                frame 6 {
                  "DT776" <- w701
                }
                frame 7 {
                }
                frame 8 {
                }
                frame 9 {
                }
              }
            }
          }
          frame "读DT32622" {
            n138 = call "读D16位.vi"("error out"=w706, "读取D地址"=32622, "VISA resource name out"=w707) -> ("error IO"=w703:errorcluster, "数值"=→"DT32622":u32, "VISA resource name out 2"=w704:refnum<visa-resource-name>)  [unwired: 5 in, 1 out]
          }
          frame "无" {
          }
          frame "读DDT32700" {
            n139 = call "读D32位.vi"("error out"=w714, "读取D地址"=32700, "VISA resource name out"=w715) -> ("error IO"=w711:errorcluster, "数值"=→"DDT32700":i32, "VISA resource name out 2"=w712:refnum<visa-resource-name>)  [unwired: 6 in]
          }
          frame "读DDT32750+10" {
            n140 = call "批量读D+5个+32位.vi"("error out"=w720, "读取D地址"=32748, "VISA resource name out"=w721) -> ("error IO"=w717:errorcluster, "数组"=w716:i32[], "VISA resource name out 2"=w718:refnum<visa-resource-name>)  [unwired: 5 in, 1 out]
            n141 = for {
              tunnel: w716 -> [w722] mode=indexing
              i -> [w723]
              n142 = case shown="0, 默认" w723 {
                tunnel: w722 -> [w724 w725 _ _ _]
                frame 0, Default {
                  "DDT32748" <- w724
                }
                frame 1 {
                  "DDT32750" <- w725
                }
                frame 2 {
                }
                frame 3 {
                }
                frame 4 {
                }
              }
            }
          }
          frame "读DT670+10" {
            n143 = call "批量读D+10个+16位.vi"("error out"=w730, "读取D地址"=670, "VISA resource name out"=w731) -> ("error IO"=w727:errorcluster, "数组"=w726:i32[], "VISA resource name out 2"=w728:refnum<visa-resource-name>)  [unwired: 5 in, 1 out]
            n144 = for {
              tunnel: w726 -> [w732] mode=indexing
              i -> [w733]
              n145 = case shown="0, 默认" w733 {
                tunnel: w732 -> [w734 _ _ _ _ _ w735 _ _ _]
                frame 0, Default {
                  "DT670" <- w734
                }
                frame 1 {
                }
                frame 2 {
                }
                frame 3 {
                }
                frame 4 {
                }
                frame 5 {
                }
                frame 6 {
                  "DT676" <- w735
                }
                frame 7 {
                }
                frame 8 {
                }
                frame 9 {
                }
              }
            }
          }
          frame "读DT660+10" {
            n146 = call "批量读D+10个+16位.vi"("error out"=w740, "读取D地址"=660, "VISA resource name out"=w741) -> ("error IO"=w737:errorcluster, "数组"=w736:i32[], "VISA resource name out 2"=w738:refnum<visa-resource-name>)  [unwired: 5 in, 1 out]
            n147 = for {
              tunnel: w736 -> [w742] mode=indexing
              i -> [w743]
              n148 = case shown="6" w743 {
                tunnel: w742 -> [w744 _ _ _ _ _ w745 _ _ _]
                frame 0, Default {
                  "DT660" <- w744
                }
                frame 1 {
                }
                frame 2 {
                }
                frame 3 {
                }
                frame 4 {
                }
                frame 5 {
                }
                frame 6 {
                  "DT666" <- w745
                }
                frame 7 {
                }
                frame 8 {
                }
                frame 9 {
                }
              }
            }
          }
          frame "读DDT600+10" {
            n149 = call "批量读D+5个+32位.vi"("error out"=w750, "读取D地址"=600, "VISA resource name out"=w751) -> ("error IO"=w748:errorcluster, "数组"=w747:i32[], "VISA resource name out 2"=w749:refnum<visa-resource-name>)  [unwired: 5 in, 1 out]
            n150 = for {
              tunnel: w747 -> [w752] mode=indexing
              i -> [w753]
              n151 = case shown="0, 默认" w753 {
                tunnel: w752 -> [w754 _ w755 _ _]
                frame 0, Default {
                  "DDT600" <- w754
                }
                frame 1 {
                }
                frame 2 {
                  "DDT604" <- w755
                }
                frame 3 {
                }
                frame 4 {
                }
              }
            }
          }
          frame "读DDT590+10" {
            n152 = call "批量读D+5个+32位.vi"("error out"=w760, "读取D地址"=590, "VISA resource name out"=w761) -> ("error IO"=w757:errorcluster, "数组"=w756:i32[], "VISA resource name out 2"=w758:refnum<visa-resource-name>)  [unwired: 5 in, 1 out]
            n153 = for {
              tunnel: w756 -> [w763] mode=indexing
              i -> [w762]
              n154 = case shown="0, 默认" w762 {
                tunnel: w763 -> [w764 _ w765 _ _]
                frame 0, Default {
                  "DDT590" <- w764
                }
                frame 1 {
                }
                frame 2 {
                  "DDT594" <- w765
                }
                frame 3 {
                }
                frame 4 {
                }
              }
            }
          }
          frame "读DDT90348" {
            n155 = call "批量读D+5个+32位.vi"("error out"=w776, "读取D地址"=90348, "VISA resource name out"=w777) -> ("error IO"=w774:errorcluster, "数组"=w781:i32[], "VISA resource name out 2"=w775:refnum<visa-resource-name>)  [unwired: 5 in, 1 out]
            n156 = Index Array(array=w781, index #1=0 ("索引"), index #2=2 ("索引")) -> (element #1=w773:i32, element #2=w772:i32)
            n157 = To Double Precision Float(number=w772) -> (double precision float=w767:dbl)
            n158 = To Double Precision Float(number=w773) -> (double precision float=w771:dbl)
            n159 = Divide(x=w767, y=100.0) -> (x/y=→"DDT90352":dbl)
            n160 = Divide(x=w771, y=100.0) -> (x/y=→"DDT90348":dbl)
          }
          frame "" {
            n161 = local read "毫秒计时值"() -> (w785:u32)
            n162 = Tick Count (ms)() -> (millisecond timer value=w786:u32)
            n163 = Subtract(x=w786, y=w785) -> (x-y=w784:u32)
            n164 = Divide(x=w784, y=u32 1000) -> (x/y=→"通讯周期":dbl)
          }
        }
        n165 = case shown="假" w58 {
          tunnel: w57 -> [w68 _]
          tunnel: [w67 _] -> w56
          frame False {
            n166 = Increment(x=w68) -> (x+1=w67:T1)
          }
          frame True {
          }
        }
        n167 = call "字符串入队列操作.vi"("字符消息入队列"="读", "界面切换队列"=w59) -> ()  [unwired: 9 in, 1 out]
      }
      frame "写" {
        n168 = call "状态匹配.vi"("输入状态"=w792) -> ("输出状态"=w791:string)  [unwired: 10 in]
        n169 = case shown="\"\", 默认" w791 {
          selector: w791 -> [w803 _ _ _ _]
          tunnel: w800 -> [_ _ _ _ w847]
          tunnel: w799 -> [_ w809 w826 _ _]
          tunnel: w798 -> [_ _ _ w837 _]
          tunnel: w797 -> [w802 w819 w830 w842 w846]
          tunnel: w796 -> [w801 w818 w829 w841 w845]
          tunnel: [_ _ _ _ TRUE] -> w795
          tunnel: [w802 w817 w828 w840 w846] -> w794
          tunnel: [w801 w816 w827 w839 w845] -> w793
          tunnel: w792 -> [_ w808 w820 w831 _]
          tunnel: [_ _ _ _ TRUE ("元素")] -> w790
          frame "", Default {
            n170 = Concatenate Strings("无对应消息分支**" ("消息"), w803, "**" ("字符串"), "写状态机" ("字符串")) -> (w807:string)
            n171 = One Button Dialog(message=w807) -> ()  [unwired: 1 in, 1 out]
          }
          frame "写DT" {
            n172 = String Length(string=w808) -> (length=w814:i32)
            n173 = Subtract(x=w814, y=4) -> (x-y=w812:i32)
            n174 = String Subset(string=w808, offset (0)=4 ("偏移量(0)"), length (rest)=w812) -> (substring=w811:string)
            n175 = Decimal String To Number(string=w811) -> (number=w810:i32)  [unwired: 2 in, 1 out]
            n176 = call "写D+16位.vi"("error out"=w818, "输入数值"=w809, "输入地址D"=w810, "VISA resource name out"=w819) -> ("error out 2"=w816:errorcluster, "VISA resource name out 2"=w817:refnum<visa-resource-name>)  [unwired: 3 in, 3 out]
          }
          frame "写DDT" {
            n177 = String Length(string=w820) -> (length=w824:i32)
            n178 = Subtract(x=w824, y=5) -> ()  [unwired: 1 out]
            n179 = String Subset(string=w820, offset (0)=5 ("偏移量(0)")) -> (substring=w821:string)  [unwired: 1 in]
            n180 = Decimal String To Number(string=w821) -> (number=w822:i32)  [unwired: 2 in, 1 out]
            n181 = call "写D+32位.vi"("error out"=w829, "输入数值"=w826, "输入地址D"=w822, "VISA resource name out"=w830) -> ("error out 2"=w827:errorcluster, "VISA resource name out 2"=w828:refnum<visa-resource-name>)  [unwired: 4 in, 2 out]
          }
          frame "写R" {
            n182 = String Length(string=w831) -> (length=w835:i32)
            n183 = Subtract(x=w835, y=3) -> (x-y=w833:i32)
            n184 = String Subset(string=w831, offset (0)=3 ("偏移量(0)"), length (rest)=w833) -> (substring=w832:string)
            n185 = call "写触点.vi"("布尔"=w837, "error out"=w841, "触点类型"="R", "写入起始地址"=w832, "VISA resource name out"=w842) -> ("error IO"=w839:errorcluster, "VISA resource name out 2"=w840:refnum<visa-resource-name>)  [unwired: 4 in, 1 out]
          }
          frame "写退出" {
            n186 = Flush Queue(queue=w847) -> (queue out=w848:refnum<queue>, error out=w849:errorcluster)  [unwired: 1 in, 1 out]
            n187 = Release Queue(queue=w848, error in (no error)=w849) -> ()  [unwired: 1 in, 3 out]
          }
        }
      }
    }
    n188 = Format Date/Time String(time format string (%c)="%A" ("时间格式字符串(%c)")) -> (date/time string=w28:string)  [unwired: 2 in]
    n189 = Get Date/Time String(date format (0)=enum16{"short", "long", "abbreviated"}."abbreviated" ("日期格式(0)"), want seconds? (F)=TRUE ("需要秒？(F)")) -> (date string=w45:string, time string=w26:string)  [unwired: 1 in]
    n190 = Concatenate Strings(w45, w27, w28, w27, w26) -> (→"字符串":string)
    n191 = Enqueue Element(queue=w23, element=w24) -> ()  [unwired: 2 in, 3 out]
  }
  n192 = while {
    shift-right: [w853] -> _
    shift-left: enum16{"初始化"}."初始化" -> [w854]
    tunnel: w6 -> [w852]
    tunnel: [w850] -> w5
    stop <- w851 stop-if-true
    n193 = Dequeue Element(queue=w852) -> (queue out=w850:refnum<queue>, element=w851:bool)  [unwired: 2 in, 2 out]
    n194 = case shown="\"初始化\", 默认" w854 {
      tunnel: [enum16{"初始化"}."初始化"] -> w853
      frame "初始化", Default {
        n195 = local read "写R2+读R3"() -> (w855:bool)
        n196 = case shown="假" w855 {
          frame False {
            n197 = stacked-sequence {
              tunnel: T3."Enabled" ("禁用") -> [w858 w859 w860 w861 w862 w863 w864 w865 _ _ w866]
              frame #0 {
                n198 = property on="R75" class="Bool"("DisabledEnum"=w858) -> ()  [unwired: 2 in, 2 out]
              }
              frame #1 {
                n199 = property on="R76" class="Bool"("DisabledEnum"=w859) -> ()  [unwired: 2 in, 2 out]
              }
              frame #2 {
                n200 = property on="DT660" class="DigNum (严格)"("DisabledEnum"=w860) -> ()  [unwired: 2 in, 2 out]
              }
              frame #3 {
                n201 = property on="DT670" class="DigNum (严格)"("DisabledEnum"=w861) -> ()  [unwired: 2 in, 2 out]
              }
              frame #4 {
                n202 = property on="DT666" class="DigNum (严格)"("DisabledEnum"=w862) -> ()  [unwired: 2 in, 2 out]
              }
              frame #5 {
                n203 = property on="DT676" class="DigNum (严格)"("DisabledEnum"=w863) -> ()  [unwired: 2 in, 2 out]
              }
              frame #6 {
                n204 = property on="DT770" class="DigNum (严格)"("DisabledEnum"=w864) -> ()  [unwired: 2 in, 2 out]
              }
              frame #7 {
                n205 = property on="DT776" class="DigNum (严格)"("DisabledEnum"=w865) -> ()  [unwired: 2 in, 2 out]
              }
              frame #8 {
              }
              frame #9 {
              }
              frame #10 {
                n206 = property on="R77" class="Bool"("DisabledEnum"=w866) -> ()  [unwired: 2 in, 2 out]
              }
            }
          }
          frame True {
            n207 = stacked-sequence {
              tunnel: T3."Disabled and Grayed Out" ("禁用") -> [w868 w869 w870 w871 w872 w873 w874 w875 _ _ w876]
              frame #0 {
                n208 = property on="R75" class="Bool"("DisabledEnum"=w868) -> ()  [unwired: 2 in, 2 out]
              }
              frame #1 {
                n209 = property on="R76" class="Bool"("DisabledEnum"=w869) -> ()  [unwired: 2 in, 2 out]
              }
              frame #2 {
                n210 = property on="DT660" class="DigNum (严格)"("DisabledEnum"=w870) -> ()  [unwired: 2 in, 2 out]
              }
              frame #3 {
                n211 = property on="DT670" class="DigNum (严格)"("DisabledEnum"=w871) -> ()  [unwired: 2 in, 2 out]
              }
              frame #4 {
                n212 = property on="DT666" class="DigNum (严格)"("DisabledEnum"=w872) -> ()  [unwired: 2 in, 2 out]
              }
              frame #5 {
                n213 = property on="DT676" class="DigNum (严格)"("DisabledEnum"=w873) -> ()  [unwired: 2 in, 2 out]
              }
              frame #6 {
                n214 = property on="DT770" class="DigNum (严格)"("DisabledEnum"=w874) -> ()  [unwired: 2 in, 2 out]
              }
              frame #7 {
                n215 = property on="DT776" class="DigNum (严格)"("DisabledEnum"=w875) -> ()  [unwired: 2 in, 2 out]
              }
              frame #8 {
              }
              frame #9 {
              }
              frame #10 {
                n216 = property on="R77" class="Bool"("DisabledEnum"=w876) -> ()  [unwired: 2 in, 2 out]
              }
            }
          }
        }
        n217 = disable-structure shown="启用" {
          frame Disabled {
            n218 = call "报警信息插入.vi"() -> ()  [unwired: 7 in, 1 out]
            n219 = call "报警信息插入.vi"() -> ()  [unwired: 7 in, 1 out]
            n220 = call "报警信息插入.vi"() -> ()  [unwired: 7 in, 1 out]
            n221 = call "报警信息插入.vi"() -> ()  [unwired: 7 in, 1 out]
            n222 = call "报警信息插入.vi"() -> ()  [unwired: 7 in, 1 out]
          }
          frame Enabled {
          }
        }
      }
    }
  }
  n223 = while {
    tunnel: w2 -> [w878]
    tunnel: "界面切换队列" -> [w877]
    stop <- w879 stop-if-true
    # "38按下 43释放"
    n224 = event shown="[24] \"写R87\": 鼠标按下" {
      selector: _ -> [_ _ _ _ _ _ _ _ _ _ _ _ _ _ _ _ _ _ _ _ _ _ _ _ _ _ _ _ _ _]
      dyn-events: _ -> [_ _ _ _ _ _ _ _ _ _ _ _ _ _ _ _ _ _ _ _ _ _ _ _ _ _ _ _ _ _]
      timeout: _ -> [_ _ _ _ _ _ _ _ _ _ _ _ _ _ _ _ _ _ _ _ _ _ _ _ _ _ _ _ _ _]
      tunnel: [_ _ _ _ _ _ _ _ _ _ w960 _ _ _ w995 w1000 w1005 _ _ _ _ _ _ _ _ _ _ w1063 _ w1070] -> w879
      tunnel: w878 -> [w880 w898 w899 w911 w925 w932 w939 w945 w952 w959 w964 w966 w975 w986 w999 w1004 w1009 w1013 w1017 w1021 w1025 w1029 w1033 w1037 w1039 w1058 w1062 w1067 _ w1069]
      tunnel: w877 -> [_ _ _ _ _ _ _ _ _ _ w963 _ _ _ w998 w1003 w1008 _ _ _ _ _ _ _ _ _ _ w1066 _ w1068]
      event "DDT32700": Mouse Down {
        n225 = event-data() -> ("CtlRef"=w881:refnum<vi>)  [unwired: 1 in, 7 out]
        n226 = Two Button Dialog(message="确定清零NG产量？" ("消息")) -> (T button?=w882:bool)  [unwired: 2 in]
        n227 = case shown="真" w882 {
          tunnel: w881 -> [_ w887]
          tunnel: w880 -> [_ w891]
          frame False {
          }
          frame True {
            n228 = call "布尔复位型入队.vi"("队列输入"=w891, "数值"=38, "控件引用"=w887, "字符消息入队列"="写R71") -> ("队列输出"=w889:refnum<queue>, "控件引用 2"=w885:refnum<vi>, "字符消息出队列"=w884:string)  [unwired: 2 in]
            n229 = call "布尔复位型入队.vi"("队列输入"=w889, "数值"=43, "控件引用"=w885, "字符消息入队列"=w884) -> ()  [unwired: 2 in, 3 out]
          }
        }
      }
      event "DDT32748": Mouse Down {
        w897 = "写DDT32748" ("字符消息入队列")
        n230 = event-data() -> ("CtlRef"=w892:refnum<vi>)  [unwired: 1 in, 7 out]
        n231 = call "数值输入窗口.vi"("消息入队"=w898, "字符串"=w897, "字符消息入队列"=w897, "输入下限"=1.0, "输入上限"=9999999.0, "转换比例"=u32 1, "数据类型"=enum16{"32位", "16位"}."32位", "控件引用"=w892) -> ()  [unwired: 5 in, 3 out]
      }
      event "DDT32750": Mouse Down {
        n232 = event-data() -> ("CtlRef"=w900:refnum<vi>)  [unwired: 1 in, 7 out]
        n233 = Two Button Dialog(message="确定清零当前产量？" ("消息")) -> (T button?=w901:bool)  [unwired: 2 in]
        n234 = case shown="假" w901 {
          tunnel: w900 -> [_ w909]
          tunnel: w899 -> [_ w906]
          frame False {
          }
          frame True {
            n235 = call "布尔复位型入队.vi"("队列输入"=w906, "数值"=38, "控件引用"=w909, "字符消息入队列"="写R70") -> ("队列输出"=w910:refnum<queue>, "控件引用 2"=w904:refnum<vi>, "字符消息出队列"=w903:string)  [unwired: 2 in]
            n236 = call "布尔复位型入队.vi"("队列输入"=w910, "数值"=43, "控件引用"=w904, "字符消息入队列"=w903) -> ()  [unwired: 2 in, 3 out]
          }
        }
      }
      event "DDT594": Mouse Down {
        n237 = event-data() -> ("CtlRef"=w912:refnum<vi>)  [unwired: 1 in, 7 out]
        n238 = Two Button Dialog(message="确定清零主料盘已放次数？" ("消息")) -> (T button?=w913:bool)  [unwired: 2 in]
        n239 = case shown="真" w913 {
          tunnel: w912 -> [_ w917]
          tunnel: w911 -> [_ w918]
          frame False {
          }
          frame True {
            n240 = call "布尔复位型入队.vi"("队列输入"=w918, "数值"=0, "控件引用"=w917, "字符消息入队列"="写R73") -> ()  [unwired: 2 in, 3 out]
          }
        }
      }
      event "DT660": Mouse Down {
        w919 = "写DT660" ("字符消息入队列")
        n241 = event-data() -> ("CtlRef"=w920:refnum<vi>)  [unwired: 1 in, 7 out]
        n242 = call "数值输入窗口.vi"("消息入队"=w925, "字符串"=w919, "字符消息入队列"=w919, "输入下限"=1.0, "输入上限"=99.0, "转换比例"=u32 1, "数据类型"=enum16{"32位", "16位"}."16位", "控件引用"=w920) -> ()  [unwired: 5 in, 3 out]
      }
      event "DT666": Mouse Down {
        w926 = "写DT666" ("字符消息入队列")
        n243 = event-data() -> ("CtlRef"=w927:refnum<vi>)  [unwired: 1 in, 7 out]
        n244 = call "数值输入窗口.vi"("消息入队"=w932, "字符串"=w926, "字符消息入队列"=w926, "输入下限"=1.0, "输入上限"=99.0, "转换比例"=u32 1, "数据类型"=enum16{"32位", "16位"}."16位", "控件引用"=w927) -> ()  [unwired: 5 in, 3 out]
      }
      event "DT670": Mouse Down {
        w933 = "写DT670" ("字符消息入队列")
        n245 = event-data() -> ("CtlRef"=w934:refnum<vi>)  [unwired: 1 in, 7 out]
        n246 = call "数值输入窗口.vi"("消息入队"=w939, "字符串"=w933, "字符消息入队列"=w933, "输入下限"=1.0, "输入上限"=99.0, "转换比例"=u32 1, "数据类型"=enum16{"32位", "16位"}."16位", "控件引用"=w934) -> ()  [unwired: 5 in, 3 out]
      }
      event "DT676": Mouse Down {
        w941 = "写DT676" ("字符消息入队列")
        n247 = event-data() -> ("CtlRef"=w940:refnum<vi>)  [unwired: 1 in, 7 out]
        n248 = call "数值输入窗口.vi"("消息入队"=w945, "字符串"=w941, "字符消息入队列"=w941, "输入下限"=1.0, "输入上限"=99.0, "转换比例"=u32 1, "控件引用"=w940) -> ()  [unwired: 6 in, 3 out]
      }
      event "DT770": Mouse Down {
        w946 = "写DT770" ("字符消息入队列")
        n249 = event-data() -> ("CtlRef"=w947:refnum<vi>)  [unwired: 1 in, 7 out]
        n250 = call "数值输入窗口.vi"("消息入队"=w952, "字符串"=w946, "字符消息入队列"=w946, "输入下限"=1.0, "输入上限"=99.0, "转换比例"=u32 1, "数据类型"=enum16{"32位", "16位"}."16位", "控件引用"=w947) -> ()  [unwired: 5 in, 3 out]
      }
      event "DT776": Mouse Down {
        w953 = "写DT776" ("字符消息入队列")
        n251 = event-data() -> ("CtlRef"=w958:refnum<vi>)  [unwired: 1 in, 7 out]
        n252 = call "数值输入窗口.vi"("消息入队"=w959, "字符串"=w953, "字符消息入队列"=w953, "输入下限"=1.0, "输入上限"=99.0, "转换比例"=u32 1, "数据类型"=enum16{"32位", "16位"}."16位", "控件引用"=w958) -> ()  [unwired: 5 in, 3 out]
      }
      event "IO界面": Mouse Down {
        n253 = event-data() -> ("CtlRef"=w962:refnum<vi>)  [unwired: 1 in, 7 out]
        n254 = call "界面切换.vi"("界面切换队列输入"=w963, "切换界面名称输入"="IO界面", "Bool引用句柄"=w962, "状态转移输入"=w964) -> ("布尔"=w960:bool)  [unwired: 7 in]
      }
      event "R75": Mouse Down {
        n255 = event-data() -> ("CtlRef"=w965:refnum<vi>)  [unwired: 1 in, 7 out]
        n256 = Two Button Dialog(message="确定修改主料盘？" ("消息")) -> (T button?=w967:bool)  [unwired: 2 in]
        n257 = case shown="真" w967 {
          tunnel: w966 -> [_ w974]
          tunnel: w965 -> [_ w971]
          frame False {
          }
          frame True {
            w969 = "写R75" ("字符消息入队列")
            n258 = call "布尔复位型入队.vi"("队列输入"=w974, "数值"=38, "控件引用"=w971, "字符消息入队列"=w969) -> ("队列输出"=w972:refnum<queue>)  [unwired: 2 in, 2 out]
            n259 = call "布尔复位型入队.vi"("队列输入"=w972, "数值"=43, "控件引用"=w971, "字符消息入队列"=w969) -> ()  [unwired: 2 in, 3 out]
          }
        }
      }
      event "R76": Mouse Down {
        n260 = event-data() -> ("CtlRef"=w976:refnum<vi>)  [unwired: 1 in, 7 out]
        n261 = Two Button Dialog(message="确定修改备料盘？" ("消息")) -> (T button?=w977:bool)  [unwired: 2 in]
        n262 = case shown="真" w977 {
          tunnel: w976 -> [_ w979]
          tunnel: w975 -> [_ w980]
          frame False {
          }
          frame True {
            w981 = "写R76" ("字符消息入队列")
            n263 = call "布尔复位型入队.vi"("队列输入"=w980, "数值"=38, "控件引用"=w979, "字符消息入队列"=w981) -> ("队列输出"=w983:refnum<queue>)  [unwired: 2 in, 2 out]
            n264 = call "布尔复位型入队.vi"("队列输入"=w983, "数值"=43, "控件引用"=w979, "字符消息入队列"=w981) -> ()  [unwired: 2 in, 3 out]
          }
        }
      }
      event "R77": Mouse Down {
        n265 = event-data() -> ("CtlRef"=w985:refnum<vi>)  [unwired: 1 in, 7 out]
        n266 = Two Button Dialog(message="确定修废料盘？" ("消息")) -> (T button?=w987:bool)  [unwired: 2 in]
        n267 = case shown="真" w987 {
          tunnel: w986 -> [_ w990]
          tunnel: w985 -> [_ w989]
          frame False {
          }
          frame True {
            w991 = "写R77" ("字符消息入队列")
            n268 = call "布尔复位型入队.vi"("队列输入"=w990, "数值"=38, "控件引用"=w989, "字符消息入队列"=w991) -> ("队列输出"=w993:refnum<queue>)  [unwired: 2 in, 2 out]
            n269 = call "布尔复位型入队.vi"("队列输入"=w993, "数值"=43, "控件引用"=w989, "字符消息入队列"=w991) -> ()  [unwired: 2 in, 3 out]
          }
        }
      }
      event "参数界面": Mouse Down {
        n270 = event-data() -> ("CtlRef"=w997:refnum<vi>)  [unwired: 1 in, 7 out]
        n271 = call "界面切换.vi"("界面切换队列输入"=w998, "切换界面名称输入"="参数界面", "Bool引用句柄"=w997, "状态转移输入"=w999) -> ("布尔"=w995:bool)  [unwired: 7 in]
      }
      event "产品界面": Mouse Down {
        n272 = event-data() -> ("CtlRef"=w1002:refnum<vi>)  [unwired: 1 in, 7 out]
        n273 = call "界面切换.vi"("界面切换队列输入"=w1003, "切换界面名称输入"="产品界面", "Bool引用句柄"=w1002, "状态转移输入"=w1004) -> ("布尔"=w1000:bool)  [unwired: 7 in]
      }
      event "手动界面": Mouse Down {
        n274 = event-data() -> ("CtlRef"=w1007:refnum<vi>)  [unwired: 1 in, 7 out]
        n275 = call "界面切换.vi"("界面切换队列输入"=w1008, "切换界面名称输入"="手动界面", "Bool引用句柄"=w1007, "状态转移输入"=w1009) -> ("布尔"=w1005:bool)  [unwired: 7 in]
      }
      event "写R2+读R3": Mouse Down; "写R2+读R3": Mouse Up {
        n276 = event-data() -> ("Type"=w1012:T5, "CtlRef"=w1011:refnum<vi>)  [unwired: 1 in, 6 out]
        n277 = call "布尔复位型入队.vi"("队列输入"=w1013, "数值"=w1012, "控件引用"=w1011, "字符消息入队列"="写R2") -> ()  [unwired: 2 in, 3 out]
      }
      event "写R2490": Mouse Down {
        n278 = event-data() -> ("CtlRef"=w1016:refnum<vi>)  [unwired: 1 in, 7 out]
        n279 = call "布尔切换型入队.vi"("字符串"="写R2490", "true启用入队"=TRUE, "控件引用"=w1016, "消息入队列"=w1017) -> ()  [unwired: 8 in]
      }
      event "写R452": Mouse Down {
        n280 = event-data() -> ("CtlRef"=w1020:refnum<vi>)  [unwired: 1 in, 7 out]
        n281 = call "布尔切换型入队.vi"("字符串"="写R452", "true启用入队"=TRUE, "控件引用"=w1020, "消息入队列"=w1021) -> ()  [unwired: 8 in]
      }
      event "写R453": Mouse Down {
        n282 = event-data() -> ("CtlRef"=w1024:refnum<vi>)  [unwired: 1 in, 7 out]
        n283 = call "布尔切换型入队.vi"("字符串"="写R453", "true启用入队"=TRUE, "控件引用"=w1024, "消息入队列"=w1025) -> ()  [unwired: 8 in]
      }
      event "写R454": Mouse Down {
        n284 = event-data() -> ("CtlRef"=w1028:refnum<vi>)  [unwired: 1 in, 7 out]
        n285 = call "布尔切换型入队.vi"("字符串"="写R454", "true启用入队"=TRUE, "控件引用"=w1028, "消息入队列"=w1029) -> ()  [unwired: 8 in]
      }
      event "写R6+读R7": Mouse Down; "写R6+读R7": Mouse Up {
        n286 = event-data() -> ("Type"=w1032:T5, "CtlRef"=w1031:refnum<vi>)  [unwired: 1 in, 6 out]
        n287 = call "布尔复位型入队.vi"("队列输入"=w1033, "数值"=w1032, "控件引用"=w1031, "字符消息入队列"="写R6") -> ()  [unwired: 2 in, 3 out]
      }
      event "写R80": Mouse Down; "写R80": Mouse Up {
        n288 = event-data() -> ("Type"=w1036:T5, "CtlRef"=w1035:refnum<vi>)  [unwired: 1 in, 6 out]
        n289 = call "布尔复位型入队.vi"("队列输入"=w1037, "数值"=w1036, "控件引用"=w1035, "字符消息入队列"="写R80") -> ()  [unwired: 2 in, 3 out]
      }
      event "写R87": Mouse Down {
        n290 = event-data() -> ("CtlRef"=w1038:refnum<vi>)  [unwired: 1 in, 7 out]
        n291 = Two Button Dialog(message="确定所有数据清0？" ("消息")) -> (T button?=w1040:bool)  [unwired: 2 in]
        n292 = case shown="真" w1040 {
          tunnel: w1039 -> [_ w1050]
          tunnel: w1038 -> [_ w1043]
          frame False {
          }
          frame True {
            w1045 = "写R87" ("字符消息入队列")
            n293 = call "布尔复位型入队.vi"("队列输入"=w1050, "数值"=38, "控件引用"=w1043, "字符消息入队列"=w1045) -> ("队列输出"=w1047:refnum<queue>)  [unwired: 2 in, 2 out]
            n294 = flat-sequence {
              tunnel: w1047 -> [w1054]
              tunnel: [w1054] -> w1046
              tunnel: w1045 -> [w1053]
              tunnel: [w1053] -> w1044
              tunnel: w1043 -> [w1052]
              tunnel: [w1052] -> w1042
              frame #0 {
                n295 = Wait (ms)(milliseconds to wait=u32 10 ("等待时间（毫秒）")) -> ()  [unwired: 1 out]
              }
            }
            n296 = call "布尔复位型入队.vi"("队列输入"=w1046, "数值"=43, "控件引用"=w1042, "字符消息入队列"=w1044) -> ()  [unwired: 2 in, 3 out]
          }
        }
      }
      event "写R88+读R89": Mouse Down; "写R88+读R89": Mouse Up {
        n297 = event-data() -> ("Type"=w1057:T5, "CtlRef"=w1056:refnum<vi>)  [unwired: 1 in, 6 out]
        n298 = call "布尔复位型入队.vi"("队列输入"=w1058, "数值"=w1057, "控件引用"=w1056, "字符消息入队列"="写R88") -> ()  [unwired: 2 in, 3 out]
      }
      event "写R9+读R8": Mouse Down; "写R9+读R8": Mouse Up {
        n299 = event-data() -> ("Type"=w1061:T5, "CtlRef"=w1060:refnum<vi>)  [unwired: 1 in, 6 out]
        n300 = call "布尔复位型入队.vi"("队列输入"=w1062, "数值"=w1061, "控件引用"=w1060, "字符消息入队列"="写R9") -> ()  [unwired: 2 in, 3 out]
      }
      event "自动界面": Mouse Down {
        n301 = event-data() -> ("CtlRef"=w1065:refnum<vi>)  [unwired: 1 in, 7 out]
        n302 = call "界面切换.vi"("界面切换队列输入"=w1066, "切换界面名称输入"="自动界面", "Bool引用句柄"=w1065, "状态转移输入"=w1067) -> ("布尔"=w1063:bool)  [unwired: 7 in]
      }
      event Timeout {
        n303 = event-data() -> ()  [unwired: 1 in, 3 out]
      }
      event Panel Close? {
        n304 = event-data() -> ()  [unwired: 1 in, 4 out]
        n305 = Two Button Dialog(message="确定退出程序？" ("消息")) -> (T button?=w1071:bool)  [unwired: 2 in]
        n306 = case shown="真" w1071 {
          tunnel: [_ TRUE] -> w1070
          tunnel: w1069 -> [_ w1076]
          tunnel: w1068 -> [_ w1075]
          frame False {
          }
          frame True {
            n307 = call "字符串入队列操作.vi"("字符消息入队列"="退出", "界面切换队列"=w1075) -> ()  [unwired: 9 in, 1 out]
            n308 = call "字符串入队列操作.vi"("字符消息入队列"="写退出", "界面切换队列"=w1076) -> ()  [unwired: 9 in, 1 out]
          }
        }
        n309 = event-data("Discard?"=TRUE ("放弃？")) -> ()  [unwired: 1 in, 1 out]
      }
    }
  }
  n310 = disable-structure shown="禁用" {
    frame Disabled {
      (unwired) u32 1 ("转换比例")
      (unwired) FALSE ("忽略数值上下限")
      n311 = call "布尔切换型入队.vi"() -> ()  [unwired: 12 in]
      n312 = call "批量读D+10个+16位.vi"() -> ()  [unwired: 8 in, 4 out]
      n313 = call "批量读D+5个+32位.vi"() -> ()  [unwired: 8 in, 4 out]
      n314 = call "界面切换.vi"() -> ()  [unwired: 11 in, 1 out]
      n315 = call "读D16位.vi"() -> ()  [unwired: 8 in, 4 out]
      n316 = call "写D+32位.vi"() -> ()  [unwired: 8 in, 4 out]
      n317 = call "读D32位.vi"() -> ()  [unwired: 9 in, 3 out]
      n318 = call "读触点-8位.vi"() -> ()  [unwired: 8 in, 4 out]
      n319 = call "写触点.vi"() -> ()  [unwired: 9 in, 3 out]
      n320 = call "布尔复位型入队.vi"() -> ()  [unwired: 8 in, 2 out]
      n321 = call "数值输入窗口.vi"("输入下限"=0.0, "输入上限"=9999.0, "数据类型"=enum16{"32位", "16位"}."32位") -> ("转换比例"=w1082:u32)  [unwired: 9 in, 3 out]
      n322 = call "数值输入窗口.vi"() -> ()  [unwired: 13 in, 3 out]
      n323 = call "数值输入窗口.vi"() -> ()  [unwired: 13 in, 3 out]
      n324 = call "数值输入窗口.vi"() -> ()  [unwired: 13 in, 3 out]
      n325 = call "数值输入窗口.vi"() -> ()  [unwired: 13 in, 3 out]
      n326 = call "数值输入窗口.vi"() -> ()  [unwired: 13 in, 3 out]
    }
    frame Enabled {
    }
  }
  n327 = disable-structure shown="启用" {
    frame Disabled {
      n328 = call "读触点-8位.vi"() -> ()  [unwired: 8 in, 4 out]
      n329 = call "写D+32位.vi"() -> ()  [unwired: 8 in, 4 out]
      n330 = call "批量读D+10个+16位.vi"() -> ()  [unwired: 8 in, 4 out]
      n331 = call "写D+16位.vi"() -> ()  [unwired: 7 in, 5 out]
      n332 = call "批量读D+5个+32位.vi"() -> ()  [unwired: 8 in, 4 out]
      n333 = call "字符串入队列操作.vi"() -> ()  [unwired: 11 in, 1 out]
      n334 = call "读D16位.vi"() -> ()  [unwired: 8 in, 4 out]
      n335 = call "读D32位.vi"() -> ()  [unwired: 9 in, 3 out]
      n336 = call "写触点.vi"() -> ()  [unwired: 9 in, 3 out]
      n337 = call "写触点.vi"() -> ()  [unwired: 9 in, 3 out]
    }
    frame Enabled {
    }
  }
  n338 = disable-structure shown="启用" {
    frame Disabled {
      n339 = for {
        i -> [w1084]
        n340 = case shown="9" w1084 {
          frame 0, Default {
          }
          frame 1 {
          }
          frame 2 {
          }
          frame 3 {
          }
          frame 4 {
          }
          frame 5 {
          }
          frame 6 {
          }
          frame 7 {
          }
          frame 8 {
          }
          frame 9 {
          }
        }
      }
      n341 = for {
        i -> [w1083]
        n342 = case shown="7" w1083 {
          frame 0, Default {
          }
          frame 1 {
          }
          frame 2 {
          }
          frame 3 {
          }
          frame 4 {
          }
          frame 5 {
          }
          frame 6 {
          }
          frame 7 {
          }
        }
      }
    }
    frame Enabled {
    }
  }
  n343 = while {
    tunnel: w11 -> [w1089]
    tunnel: w10 -> [w1088]
    tunnel: w5 -> [w1086]
    stop <- TRUE stop-if-true
    n344 = control-ref of="本VI"() -> (w1085:refnum<vi>)
    n345 = Release Queue(queue=w1086) -> ()  [unwired: 2 in, 3 out]
    n346 = property on="自动界面" class="Bool"("DisabledEnum"=T3."Enabled" ("禁用")) -> ()  [unwired: 2 in, 2 out]
    n347 = invoke class="VI" method="FP.Close"(reference=w1085) -> ()  [unwired: 2 in, 3 out]
    "VISA资源名称输出" <- w1089
    "错误输出" <- w1088
  }
